vi "StartSubroutine.vi"(8 "error in (no error)":errorcluster, 11 "AutoSubroutine in":refnum<class "AutoSubroutine.lvclass">) -> (0 "error out":errorcluster, 3 "AutoSubroutine out":refnum<class "AutoSubroutine.lvclass">)   [LabVIEW 2017, in "AutoSubroutine.lvclass"]
uses:
  AutoSubroutine.lvclass
  Subsystem/GetQueueRef.ctl
  AutoSubroutine.lvclass/AutoSubroutine.ctl
  Subsystem/Subsystem.lvclass
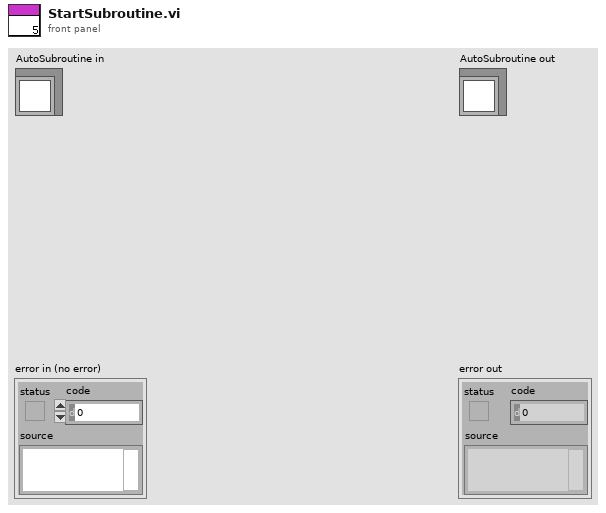
[diagram p1: front panel]
types:
  T1 = typedef "Subsystem.lvclass/GetQueueRef.ctl" = enum16{"Both", "Command", "Output"}
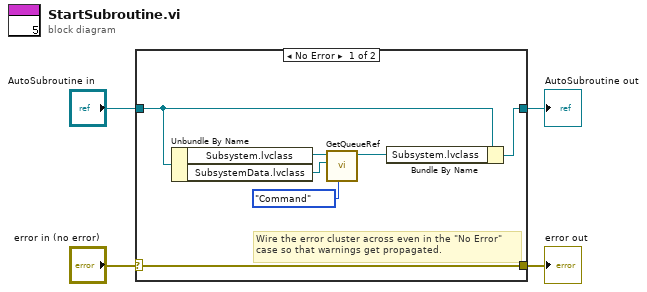
[diagram p0: block diagram]
diagram:
  n1 = case shown="No Error" "error in (no error)" {
    selector: "error in (no error)" -> [w11 w13]
    tunnel: [w11 w13] -> w3
    tunnel: [w6 w12] -> w1
    tunnel: "AutoSubroutine in" -> [w8 w12]
    frame No Error {
      # "Wire the error cluster across even in the \"No Error\"\ncase so that warnings get propagated."
      n2 = Unbundle By Name(w8) -> ("Subsystem.lvclass"=w9:refnum<class "Subsystem.lvclass">, "SubsystemData.lvclass"=w10:refnum<class "SubsystemData.lvclass">)
      n3 = call-dynamic "GetQueueRef.vi"("GetQueueRef"=GetQueueRef."Command", "SubsystemData.lvclass"=w10, "Subsystem in"=w9) -> ("Subsystem out"=w7:refnum<class "Subsystem.lvclass">)  [unwired: 7 in, 1 out]
      n4 = Bundle By Name(cluster=w8, "Subsystem.lvclass"=w7) -> (w6:refnum<class "AutoSubroutine.lvclass">)
    }
    frame Error {
    }
  }
  "error out" <- w3
  "AutoSubroutine out" <- w1
